vi "RenameTaskItem.vi"(9 "TaskConfig":refnum<data-value>, 10 "New Task":string, 11 "Old Task":string) -> ()   [LabVIEW 2025, in "DAQ_Module.lvlib" / "DAQ_Module.lvclass"]
uses:
  DAQ_Module.lvclass
  DAQ_Config.ctl
  DAQ_Task_Config.ctl
  DAQ_HW_Type.ctl
  DAQ_Task_Type.ctl
  DAQ_SampleRateConfig.ctl
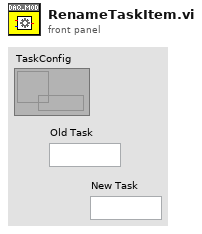
[diagram p1: front panel]
types:
  T1 = typedef "DAQ_Module.lvlib/DAQ_Module.lvclass/DAQ_Config.ctl" = map{string, T2}
  T2 = typedef "DAQ_Module.lvlib/DAQ_Module.lvclass/DAQ_Task_Config.ctl" = cluster{"Drive":T3, "TaskType":T4, "PhysicalChannels":string, "SampleRateConfiguration":T5, "ChannelConfig":map{string, cluster{"Name":string, "Config":string}}, "Enable":bool, "ShowPanel":bool}
  T3 = typedef "DAQ_Module.lvlib/DAQ_Module.lvclass/DAQ_HW_Type.ctl" = enum16{"NI_DAQmx", "Simulated_DAQ"}
  T4 = typedef "DAQ_Module.lvlib/DAQ_Module.lvclass/DAQ_Task_Type.ctl" = enum16{"AI", "Linear", "Angular", "AO"}
  T5 = typedef "DAQ_Module.lvlib/DAQ_Module.lvclass/DAQ_SampleRateConfig.ctl" = cluster{"SampleRate":dbl, "SamplesPerChannel":u32, "SamplesPerRead":i32, "SampleMode":i32, "Clock Source":string}
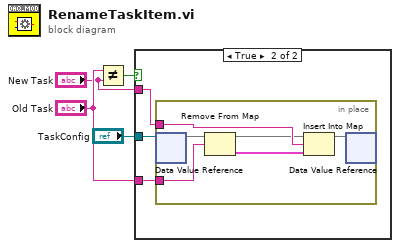
[diagram p0: block diagram]
diagram:
  n1 = Not Equal?(x="Old Task", y="New Task") -> (x != y?=w1:bool)
  n2 = case shown="True" w1 {
    tunnel: "TaskConfig" -> [_ w7]
    tunnel: "Old Task" -> [_ w6]
    tunnel: "New Task" -> [_ w5]
    frame False {
    }
    frame True {
      n3 = in-place {
        in-place-border: w6 -> [w11]
        in-place-border: w5 -> [w9]
        n4 = in-place-dvr #1(w7) -> (w12:T1)  [unwired: 1 out]
        n5 = Remove From Map(10:w11, 11:w12) -> (1:w10:T2, 3:w8:T1)  [unwired: 1 out]
        n6 = Insert Into Map(map in=w8, key=w9, value=w10) -> (map out=w13:T1)  [unwired: 2 out]
        n7 = in-place-dvr #1(w13) -> ()  [unwired: 2 out]
      }
    }
  }
